vi "Get INI Configuration.vi"(8 "error in (no error)":errorcluster, 11 "configuration file path":path) -> (0 "error out":errorcluster, 3 "INI":T1={"Library.Name"="NI VeriStand Published Data", "Alias.FolderPath"="All", "Publish.Period_ms"=0})   [LabVIEW 2013, in "Data Publishing Service.lvlib"]
uses:
  Data Publishing Service.lvlib
  Types/INI Configuration.ctl
  <vilib>/Utility/config.llb/Read Key (String).vi
  <vilib>/Utility/config.llb/Read Key (U32).vi
  <vilib>/Utility/config.llb/Write Key (String).vi
  <vilib>/Utility/config.llb/Write Key (U32).vi
  <vilib>/Utility/config.llb/NI_LVConfig.lvlib
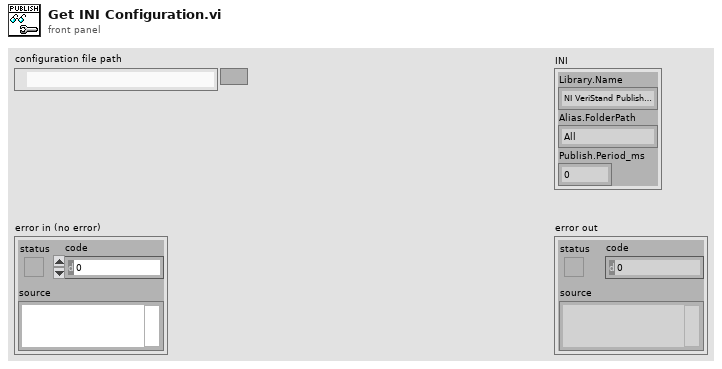
[diagram p1: front panel]
types:
  T1 = typedef "Data Publishing Service.lvlib/INI Configuration.ctl" = cluster{"Library.Name":string, "Alias.FolderPath":string, "Publish.Period_ms":u32}
  T2 = typedef "NI_LVConfig.lvlib/Config Data RefNum.ctl" = refnum<k1>
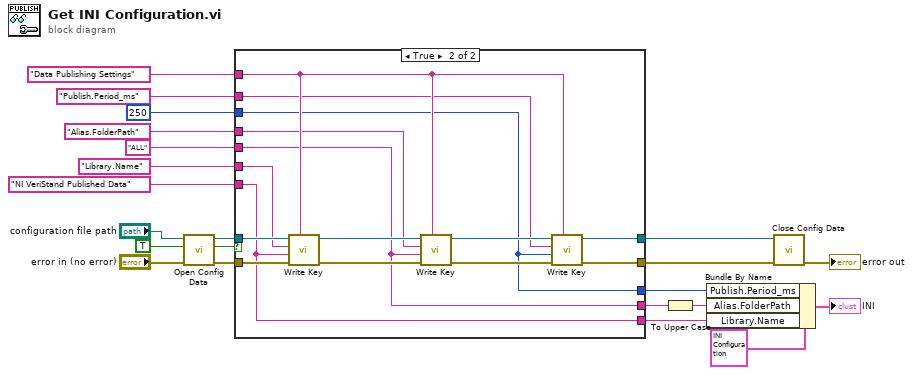
[diagram p0: block diagram]
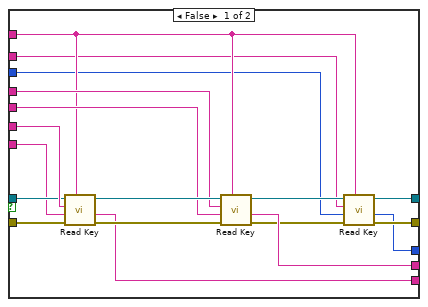
[diagram p2: hidden frame]
diagram:
  n1 = call <vilib>:"Open Config Data.vi"("error in (no error)"="error in (no error)", "create file if necessary (T)"=TRUE, "configuration file path"="configuration file path") -> ("error out"=w20:errorcluster, "file created?"=w1:bool, "refnum"=w19:T2)  [unwired: 6 in]
  n2 = case shown="True" w1 {
    tunnel: "Library.Name" ("key") -> [w40 w46]
    tunnel: w20 -> [w39 w51]
    tunnel: w19 -> [w38 w50]
    tunnel: "NI VeriStand Published Data" ("default value") -> [w37 w41]
    tunnel: "Alias.FolderPath" ("key") -> [w34 w45]
    tunnel: "ALL" ("default value") -> [w33 w42]
    tunnel: [w32 w41] -> w11
    tunnel: [w31 w42] -> w10
    tunnel: [w29 w48] -> w7
    tunnel: [w27 w49] -> w6
    tunnel: "Data Publishing Settings" ("section") -> [w26 w47]
    tunnel: "Publish.Period_ms" ("key") -> [w25 w44]
    tunnel: u32 250 ("value") -> [w24 w43]
    tunnel: [w23 w43] -> w2
    frame False {
      n3 = call-poly <vilib>:"Read Key.vi"("section"=w26, "error in (no error)"=w39, "default value"=w37, "key"=w40, "refnum"=w38) -> ("error out"=w35:errorcluster, "value"=w32:string, "refnum out"=w36:T2)  [unwired: 3 in, 1 out]
      n4 = call-poly <vilib>:"Read Key.vi"("section"=w26, "error in (no error)"=w35, "default value"=w33, "key"=w34, "refnum"=w36) -> ("error out"=w28:errorcluster, "value"=w31:string, "refnum out"=w30:T2)  [unwired: 3 in, 1 out]
      n5 = call-poly <vilib>:"Read Key.vi"("section"=w26, "error in (no error)"=w28, "default value"=w24, "key"=w25, "refnum"=w30) -> ("error out"=w27:errorcluster, "value"=w23:u32, "refnum out"=w29:T2)  [unwired: 3 in, 1 out]
    }
    frame True {
      n6 = call-poly <vilib>:"Write Key.vi"("section"=w47, "error in (no error)"=w51, "value"=w41, "key"=w46, "refnum"=w50) -> ("error out"=w53:errorcluster, "refnum out"=w52:T2)  [unwired: 4 in, 1 out]
      n7 = call-poly <vilib>:"Write Key.vi"("section"=w47, "error in (no error)"=w53, "value"=w42, "key"=w45, "refnum"=w52) -> ("error out"=w55:errorcluster, "refnum out"=w54:T2)  [unwired: 4 in, 1 out]
      n8 = call-poly <vilib>:"Write Key.vi"("section"=w47, "error in (no error)"=w55, "value"=w43, "key"=w44, "refnum"=w54) -> ("error out"=w49:errorcluster, "refnum out"=w48:T2)  [unwired: 4 in, 1 out]
    }
  }
  n9 = To Upper Case(1:w10) -> (0:w9:string)
  n10 = Bundle By Name(cluster=T1 {"Library.Name"="NI VeriStand Published Data", "Alias.FolderPath"="All", "Publish.Period_ms"=0}, "Publish.Period_ms"=w2, "Alias.FolderPath"=w9, "Library.Name"=w11) -> (→"INI":T1)
  n11 = call <vilib>:"Close Config Data.vi"("error in (no error)"=w6, "refnum"=w7) -> ("error out"=→"error out":errorcluster)  [unwired: 8 in, 1 out]
